vi "Telemetry Handler.vi"   [LabVIEW 2021]
doc: "This VI reads in all telemetry from producers and redistributes it to consumers."
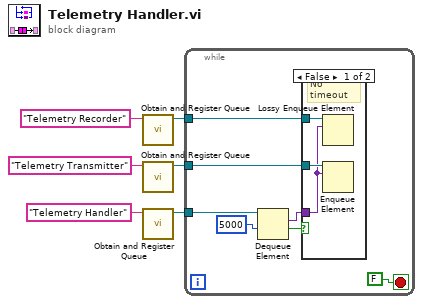
[diagram p0: block diagram]
diagram:
  n1 = call "Obtain and Register Queue.vi"("Queue Name (unnamed)"="Telemetry Recorder" ("name (unnamed)")) -> ("Queue Reference"=w1:refnum<queue>)  [unwired: 9 in, 1 out]
  n2 = call "Obtain and Register Queue.vi"("Queue Name (unnamed)"="Telemetry Transmitter" ("name (unnamed)")) -> ("Queue Reference"=w6:refnum<queue>)  [unwired: 9 in, 1 out]
  n3 = call "Obtain and Register Queue.vi"("Queue Name (unnamed)"="Telemetry Handler" ("name (unnamed)")) -> ("Queue Reference"=w3:refnum<queue>)  [unwired: 9 in, 1 out]
  n4 = while {
    tunnel: w3 -> [w13]
    tunnel: w6 -> [w11]
    tunnel: w1 -> [w10]
    stop <- FALSE stop-if-true
    n5 = Dequeue Element(queue=w13, timeout in ms (-1)=5000) -> (element=w9:variant, timed out?=w8:bool)  [unwired: 1 in, 2 out]
    n6 = case shown="False" w8 {
      tunnel: w11 -> [w16 _]
      tunnel: w10 -> [w15 _]
      tunnel: w9 -> [w14 _]
      frame False {
        # "No timeout"
        n7 = Lossy Enqueue Element(queue=w15, element=w14) -> ()  [unwired: 1 in, 4 out]
        n8 = Enqueue Element(queue=w16, element=w14) -> ()  [unwired: 2 in, 3 out]
      }
      frame True {
        # "Timed out"
      }
    }
  }
